vi "Path Manager.vi"(11 "error in (no error)":errorcluster) -> (4 "Cluster":T1, 15 "Error out":errorcluster)   [LabVIEW 2022 SP3]
uses:
  Paths.ctl
  <vilib>/Utility/sysdir.llb/System Directory Type.ctl
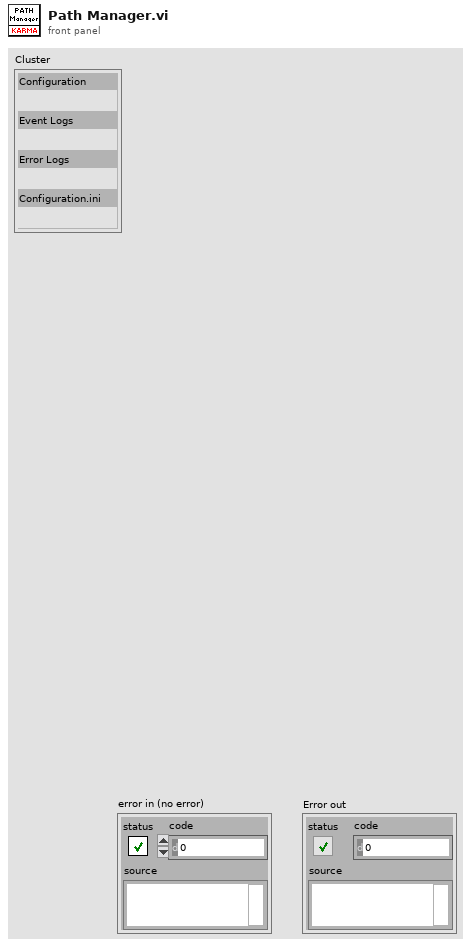
[diagram p1: front panel]
types:
  T1 = typedef "Paths.ctl" = cluster{"Configuration":path, "Event Logs":path, "Error Logs":path, "Configuration.ini":path}
  T2 = typedef "System Directory Type.ctl" = i32
  T3 = cluster{"File Array[0]":path, "File Array[1]":path, "File Array[2]":path, "File Array[3]":path, "File Array[4]":path, "File Array[5]":path, "File Array[6]":path, "File Array[7]":path, "File Array[8]":path, "File Array[9]":path}
  T4 = cluster{"File Array[0]":path, "File Array[1]":path, "File Array[2]":path, "File Array[3]":path, "File Array[4]":path, "File Array[5]":path, "File Array[6]":path, "File Array[7]":path, "File Array[8]":path}
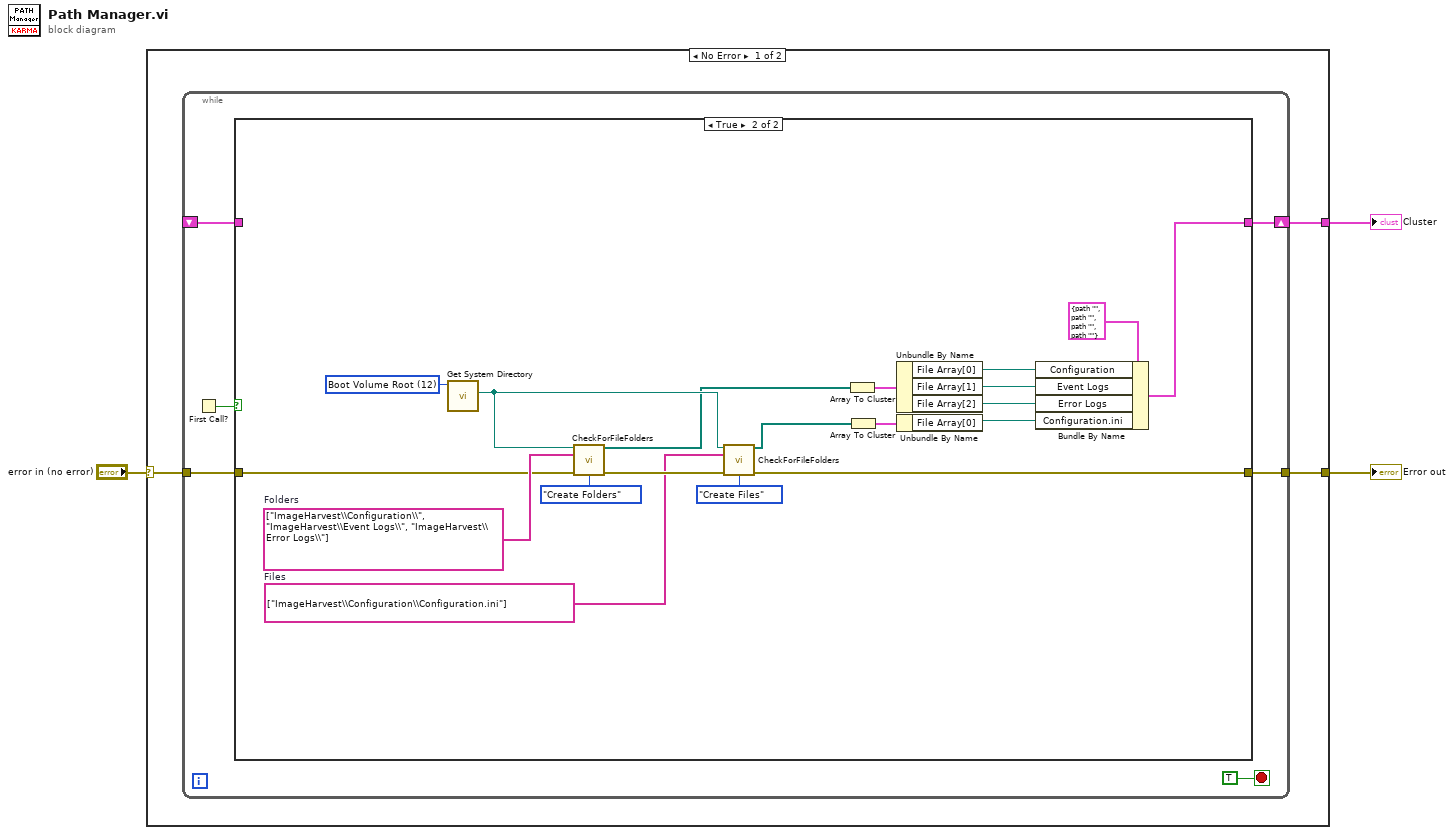
[diagram p0: block diagram]
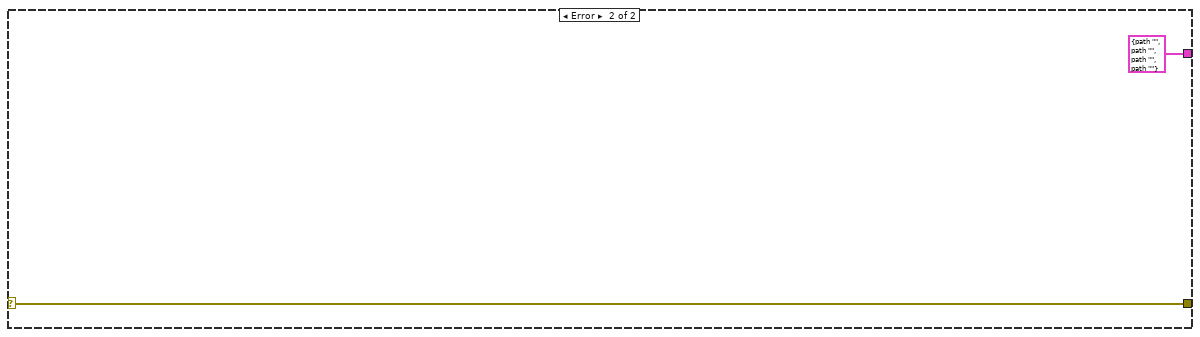
[diagram p3: hidden frame]
diagram:
  n1 = case shown="No Error" "error in (no error)" {
    selector: "error in (no error)" -> [w4 w34]
    tunnel: [w6 T1 {"Configuration"=path "", "Event Logs"=path "", "Error Logs"=path "", "Configuration.ini"=path ""}] -> w3
    tunnel: [w5 w34] -> w2
    frame No Error {
      n2 = while {
        tunnel: w4 -> [w11]
        shift-right: [w10] -> w6
        shift-left: _ -> [w8]
        tunnel: [w7] -> w5
        stop <- TRUE stop-if-true
        n3 = First Call?() -> (First Call?: T/F=w9:bool)
        n4 = case shown="True" w9 {
          tunnel: w11 -> [w13 w31]
          tunnel: [w13 w16] -> w7
          tunnel: [w14 w17] -> w10
          tunnel: w8 -> [w14 _]
          frame False {
          }
          frame True {
            w26 = string[] ["ImageHarvest\\Configuration\\Configuration.ini"]  # Files
            w32 = string[] ["ImageHarvest\\Configuration\\", "ImageHarvest\\Event Logs\\", "ImageHarvest\\Error Logs\\"]  # Folders
            w33 = T2 12 items=["User Home"=0, "User Desktop"=1, "User Documents"=2, "User Application Data"=3, "User Preferences"=4, "User Temporary"=5, "Public Documents"=6, "Public Application Data"=7, "Public Preferences"=8, "Public Cache"=13, "System Core Libraries"=9, "System Installed Libraries"=10, "Application Files"=11, "Boot Volume Root"=12] ("system directory type")
            n5 = call <vilib>:"Get System Directory.vi"("system directory type"=w33) -> ("system directory"=w27:path)  [unwired: 10 in]
            n6 = call "CheckForFileFolders.vi"("Main Path"=w27, "Sub Path"=w32, "Error in (no error)"=w31, "Operation"=enum16{"Create Files", "Create Folders"}."Create Folders") -> ("File Array"=w25:path[], "Error out"=w30:errorcluster)  [unwired: 10 in]
            n7 = call "CheckForFileFolders.vi"("Main Path"=w27, "Sub Path"=w26, "Error in (no error)"=w30, "Operation"=enum16{"Create Files", "Create Folders"}."Create Files") -> ("File Array"=w19:path[], "Error out"=w16:errorcluster)  [unwired: 10 in]
            n8 = Array To Cluster(array=w25) -> (cluster=w24:T3)
            n9 = Array To Cluster(array=w19) -> (cluster=w18:T4)
            n10 = Unbundle By Name(w24) -> ("File Array[0]"=w22:path, "File Array[1]"=w20:path, "File Array[2]"=w21:path)
            n11 = Unbundle By Name(w18) -> ("File Array[0]"=w15:path)
            n12 = Bundle By Name(cluster=T1 {"Configuration"=path "", "Event Logs"=path "", "Error Logs"=path "", "Configuration.ini"=path ""}, "Configuration"=w22, "Event Logs"=w20, "Error Logs"=w21, "Configuration.ini"=w15) -> (w17:T1)
          }
        }
      }
    }
    frame Error {
    }
  }
  "Cluster" <- w3
  "Error out" <- w2
